vi "BarcodeComplete.vi"(11 "Data In":T1) -> (1 "Complete":bool, 3 "Data Out":T1)   [LabVIEW 2014]
uses:
  controls/Data1.ctl
  controls/Payjson.ctl
panel:
  out "number":u32
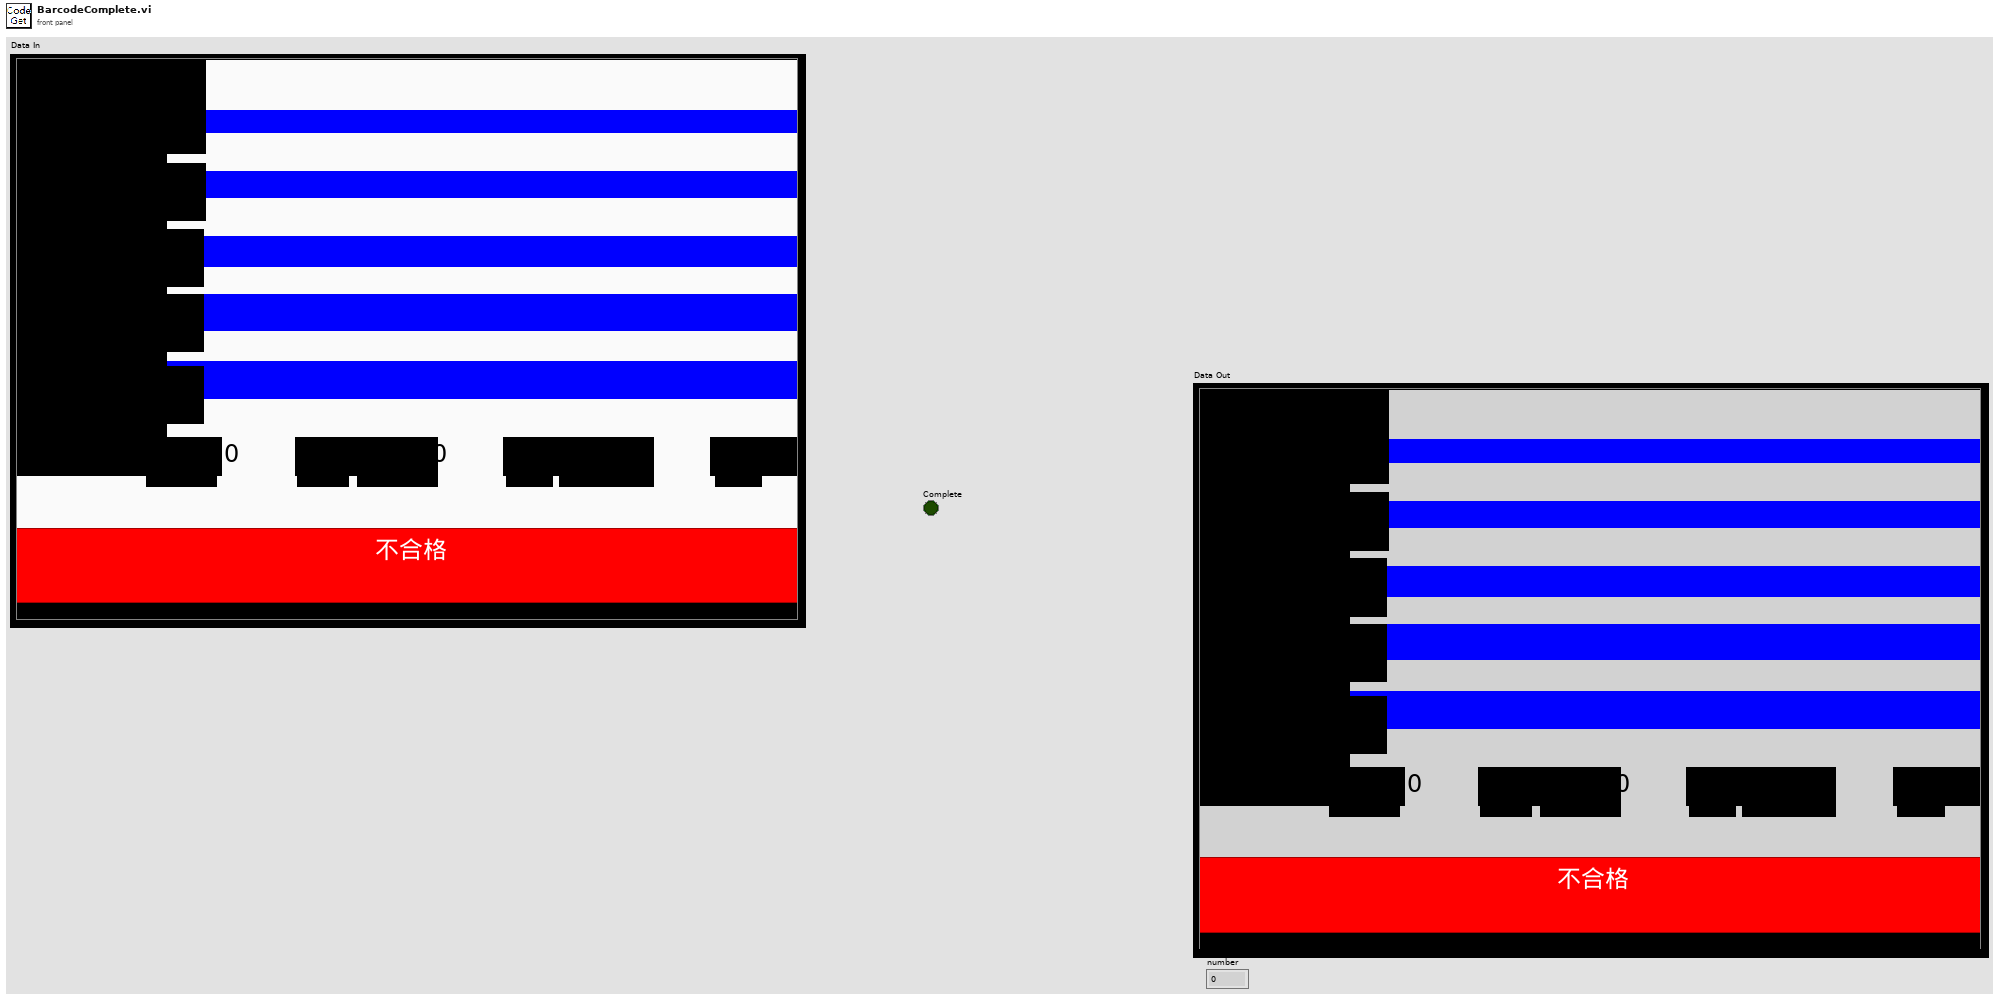
[diagram p1: front panel]
types:
  T1 = typedef "Data1.ctl" = cluster{"Date":string, "BarCode1":string, "BarCode2":string, "BarCode3":string, "Message":string, "OK Count":u16, "NG Count":u16, "Total Count":u16, "ModelData":string[][], "OK&NG":bool, "COM1":refnum<visa-resource-name>, "COM2":refnum<visa-resource-name>, "IO":i32, "Time":u32, "TCP":refnum<k5>, "TCP 2":refnum<k5>, "COM1 2":refnum<visa-resource-name>, "CheckNum":string, "BarCode1_1":string, "BarCode2_1":string, "BarCode3_1":string, "日期":string, "機種":string, "機號":string, "商品條碼1":string, "OK_1":string, "OK":string, "NG":string, "NG_1":string, "Total":string, "Total_1":string, "ClaerTime":u32, "Pjson":T2, "LotNo":string[], "CheckParsArray":string[], "BarCode4":string, "BarCode4_1":string, "商品條碼2":string, "BarCode5":string, "BarCode5_1":string, "商品條碼3":string, "ReScanNG":i32, "NGTimeCT":u32}
  T2 = typedef "Payjson.ctl" = cluster{"DEPT":string, "LINE":string, "STANO":string, "WORKNO":string, "PRODSN":string, "COMPNTID":string, "COMPNTLOT":string, "COMPNTSN":string, "USEDQTY":i16, "OPDATE":string, "OPUSER":string, "RECVDATE":string, "MMODU":string}[]
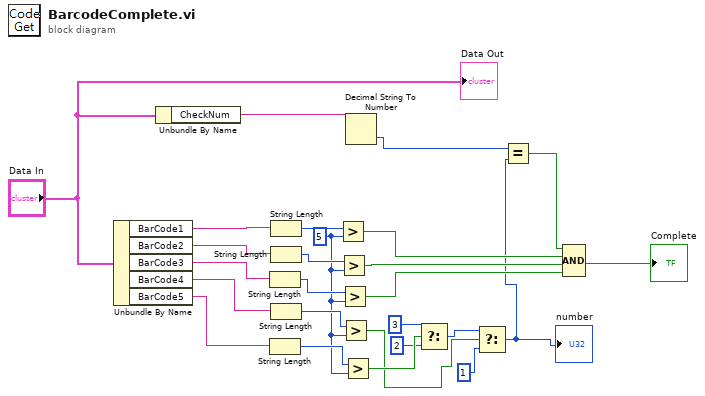
[diagram p0: block diagram]
diagram:
  w11 = 5 ("y")
  n1 = Unbundle By Name("Data In") -> ("BarCode1"=w26:string, "BarCode2"=w25:string, "BarCode3"=w24:string, "BarCode4"=w15:string, "BarCode5"=w14:string)
  n2 = Unbundle By Name("Data In") -> ("CheckNum"=w16:string)
  n3 = String Length(string=w24) -> (length=w21:i32)
  n4 = String Length(string=w14) -> (length=w12:i32)
  n5 = String Length(string=w26) -> (length=w23:i32)
  n6 = String Length(string=w25) -> (length=w22:i32)
  n7 = String Length(string=w15) -> (length=w13:i32)
  n8 = Greater?(x=w23, y=w11) -> (0:w20:bool)
  n9 = Greater?(x=w22, y=w11) -> (0:w19:bool)
  n10 = Greater?(x=w21, y=w11) -> (0:w10:bool)
  n11 = Greater?(x=w13, y=w11) -> (0:w6:bool)
  n12 = Greater?(x=w12, y=w11) -> (0:w9:bool)
  n13 = Decimal String To Number(string=w16) -> (number=w3:i32)  [unwired: 2 in, 1 out]
  n14 = Select(t=3 ("y"), s=w9, f=2) -> (s? t:f=w5:i32)
  n15 = Select(t=w5, s=w6, f=1) -> (s? t:f=w2:i32)
  "number" <- w2
  n16 = Equal?(x=w3, y=w2) -> (x = y?=w1:bool)
  n17 = Compound Arithmetic op=AND(w1, w20, w19, w10) -> (→"Complete":bool)
  "Data Out" <- "Data In"
